vi "Init.vi"(7 "Prepend Result Name":bool, 8 "error in (no error)":errorcluster, 9 "SA Pin":string, 10 "Measurement Name":string) -> (0 "error out":errorcluster, 3 "SpecAn_AMPM out":refnum<class "SpecAn_AMPM.lvclass">)   [LabVIEW 2018, in "SeqAuto Evaluations.lvlib" / "SpecAn_AMPM.lvclass"]
uses:
  SpecAn_AMPM.lvclass
  C:/Sequence Automation/Plugins/SeqAuto IEvaluation.lvlibp/SeqAuto IEvaluation.lvclass
  SpecAn_AMPM.lvclass/SpecAn_AMPM.ctl
  Write SA Pin.vi
  Plugins/SeqAuto IEvaluation.lvlibp/Write Measurement Name.vi
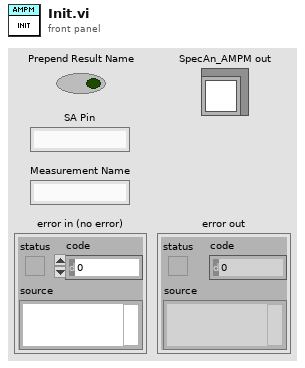
[diagram p1: front panel]
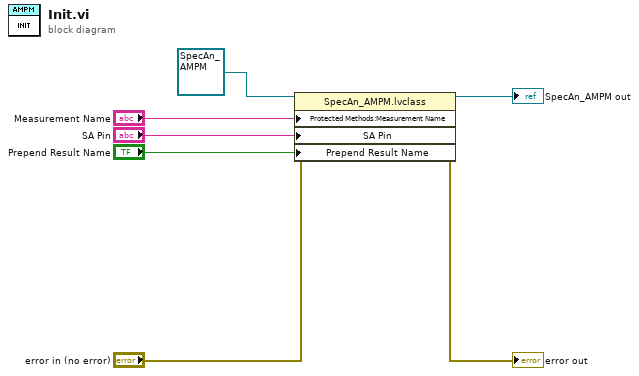
[diagram p0: block diagram]
diagram:
  n1 = property class="SpecAn_AMPM.lvclass"(reference=refnum<class "SpecAn_AMPM.lvclass"> refnum ("SpecAn_CHP in"), error in="error in (no error)", "Protected Methods:Measurement Name"="Measurement Name", "SA Pin"="SA Pin", "Prepend Result Name"="Prepend Result Name") -> (reference out=→"SpecAn_AMPM out":refnum<class "SpecAn_AMPM.lvclass">, error out=→"error out":errorcluster)
